vi "Configure Output Parameters(CM).vi"(7 "Unit Address (1)":u8=1, 8 "error in (no error)":errorcluster, 9 "Cooling Algorithm Type (0:Linear)":u8(ring) items=["Linear", "Oil", "Water", "Fan"], 10 "Power Feed Forward (False: Disable)":bool, 11 "VISA resource name":refnum<visa-resource-name>) -> (0 "error out":errorcluster, 3 "VISA resource name out":refnum<visa-resource-name>)   [LabVIEW 2014, in "Eurotherm 35xx Series.lvlib"]
doc: "This VI configure output CM (Configuration Mode) parameters.\n\nWarning: This VI uses Controller Configuration Mode, this interrupts working process (device will not control).\nIt is recommended that the device should be disconnected from any active process."
uses:
  <instrlib>/Eurotherm 35xx Series/Eurotherm 35xx Series.lvlib
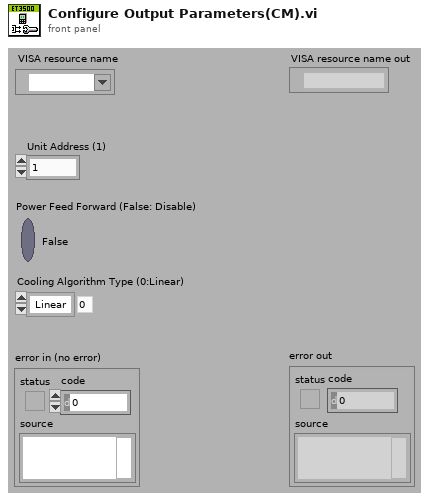
[diagram p1: front panel]
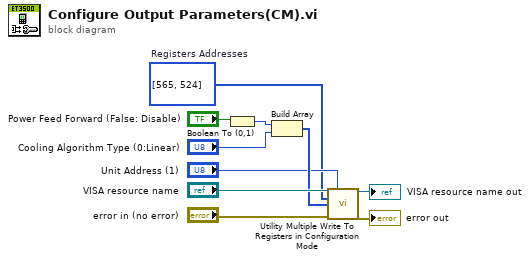
[diagram p0: block diagram]
diagram:
  w1 = u16[] [565, 524]  # Registers Addresses
  n1 = Boolean To (0,1)(Boolean="Power Feed Forward (False: Disable)") -> (0, 1=w5:i16)
  n2 = Build Array(w5, "Cooling Algorithm Type (0:Linear)") -> (w6:i16[])
  n3 = call <instrlib>:"Utility Multiple Write To Registers in Configuration Mode.vi"("VISA resource name"="VISA resource name", "Unit Address (1)"="Unit Address (1)", "Registers Addresses (0)"=w1, "Data (0)"=w6, "error in (no error)"="error in (no error)") -> ("VISA resource name out"=→"VISA resource name out":refnum<visa-resource-name>, "error out"=→"error out":errorcluster)  [unwired: 9 in]
